vi "FancyDrive.vi"(8 "Y axis value":dbl, 11 "X axis value":dbl) -> (0 "Right Motor Value":dbl, 3 "Left Motor Value":dbl)   [LabVIEW 2020]
uses:
  <vilib>/Rock Robotics/WPI/Joystick/WPI_JoystickArcadeMapping.vi
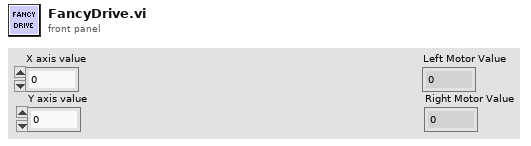
[diagram p1: front panel]
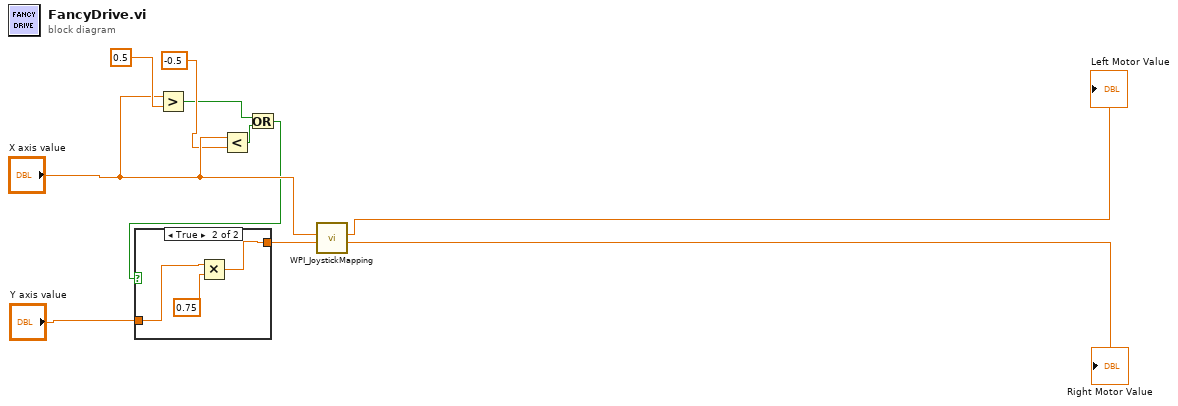
[diagram p0: block diagram]
diagram:
  n1 = Greater?(x="X axis value", y=0.5) -> (0:w3:bool)
  n2 = Less?(x="X axis value", y=-0.5) -> (x < y?=w2:bool)
  n3 = Or(x=w3, y=w2) -> (x .or. y?=w1:bool)
  n4 = case shown="True" w1 {
    tunnel: [w11 w12] -> w9
    tunnel: "Y axis value" -> [w11 w13]
    frame False {
    }
    frame True {
      n5 = Multiply(x=w13, y=0.75) -> (x*y=w12:dbl)
    }
  }
  n6 = call-poly <vilib>:"WPI_JoystickMapping.vi"("Y axis value"=w9, "X axis value"="X axis value") -> ("Right Motor Value"=→"Right Motor Value":dbl, "Left Motor Value"=→"Left Motor Value":dbl)  [unwired: 8 in]
